vi "decimal string trim end.vi"(8 "error in (no error)":errorcluster, 11 "Decimal number string":string) -> (0 "error out":errorcluster, 3 "Just decimal part":string)   [LabVIEW 2013]
doc: "Takes a decimal string and trims the end when decimal number ends"
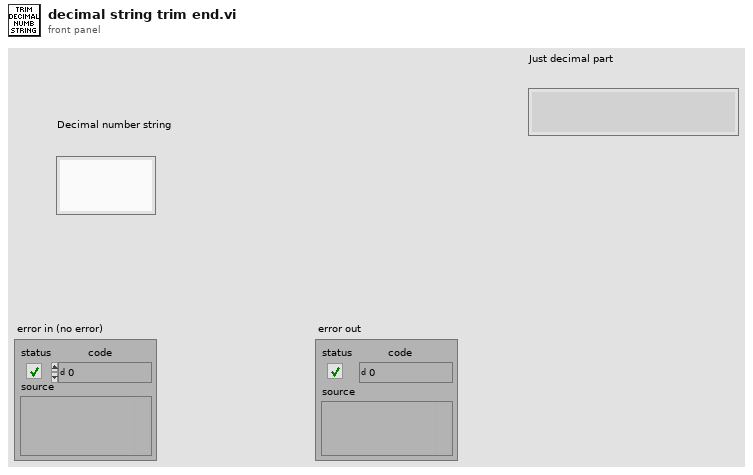
[diagram p1: front panel]
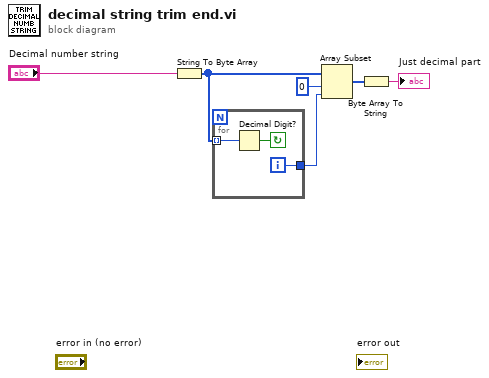
[diagram p0: block diagram]
diagram:
  n1 = String To Byte Array(string="Decimal number string") -> (unsigned byte array=w5:u8[])
  n2 = for {
    tunnel: w5 -> [w9] mode=indexing
    tunnel: [w7] -> w3
    i -> [w7]
    stop <- w8 continue-if-true
    n3 = Decimal Digit?(1:w9) -> (0:w8:bool)
  }
  n4 = Array Subset(array=w5, index=0, length=w3) -> (w2:u8[])
  n5 = Byte Array To String(unsigned byte array=w2) -> (string=→"Just decimal part":string)
